vi "get_message_type.vi"(8 "error in (no error)":errorcluster, 11 "message_text in":refnum<class "message_image.lvclass">) -> (0 "error out":errorcluster, 2 "Type":string, 3 "message_text out":refnum<class "message_image.lvclass">)   [LabVIEW 2020, in "message_image.lvclass"]
uses:
  message_image.lvclass
  abstract_message_base/abstract_message_base.lvclass
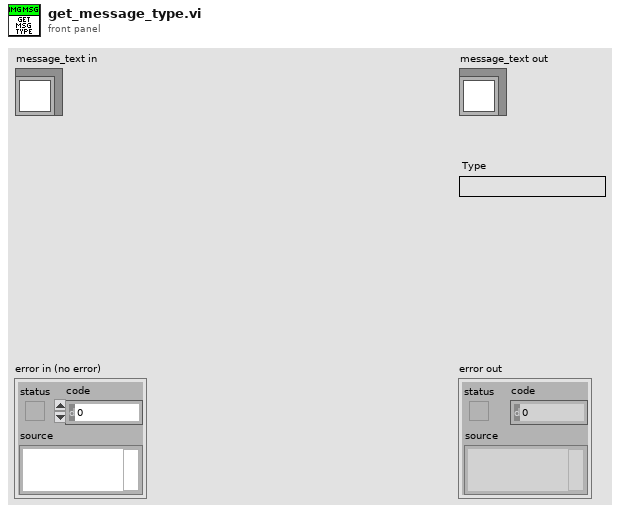
[diagram p1: front panel]
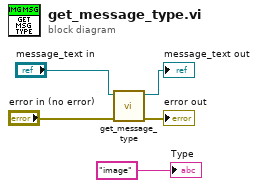
[diagram p0: block diagram]
diagram:
  n1 = call-parent "get_message_type.vi"("error in (no error)"="error in (no error)", "abstract_message_base in"="message_text in") -> ("error out"=→"error out":errorcluster, "abstract_message_base out"=→"message_text out":refnum<class "message_image.lvclass">)  [unwired: 7 in, 1 out]
  "Type" <- "image" ("Type")
